vi "Line_detector_Labview.vi"() -> ()   [LabVIEW 2021]
uses:
  <vilib>/Analysis/NI_AALPro.lvlib
  <vilib>/Analysis/8numeric.llb/1D Numeric Integration.vi
  <vilib>/Utility/file.llb/Write To Spreadsheet File (DBL).vi
panel:
  in  "length droplet 13":i32=50
  in  "start droplet 13":i32=885
  in  "length droplet 12":i32=50
  in  "start droplet 12":i32=820
  in  "Length droplet 11":i32=50
  in  "start droplet 11":i32=750
  in  "droplet length 10":i32=50
  in  "start droplet 10":i32=690
  in  "length droplet 9":i32=50
  in  "start droplet 9":i32=630
  in  "length droplet 8":i32=50
  in  "start droplet 8":i32=540
  in  "length droplet 7":i32=50
  in  "start droplet 7":i32=480
  in  "Length droplet 6":i32=50
  in  "start droplet 6":i32=420
  in  "droplet length 5":i32=50
  in  "start droplet 5":i32=380
  out "Waveform Chart":dynamicdata(graph)
  in  "length droplet 4":i32=50
  in  "start droplet 4":i32=315
  in  "length droplet 3":i32=50
  in  "start droplet 3":i32=250
  in  "Length droplet 2":i32=50
  in  "start droplet 2":i32=190
  in  "stop":bool
  in  "droplet length 1":i32=50
  in  "start droplet 1":i32=120
  out "Device Status":i32
  in  "filename":string="CCS_1"
  in  "Directory 2":path=path "C:/My_directory"
  in  "Recording time":dbl=600.0
  out "Time (s)":u32
  out "Waveform Graph":dbl[](graph)=[0.04596838682352941, 0.044503448, 0.04074093858823529, 0.042205794117647064, 0.04124974823529412, 0.03858205317647059, 0.037749302352941175, 0.03488108894117647, 0.033539547999999995, 0.03310773858823529, 0.03099518376470588, 0.03062508070588235, 0.029792362823529414, 0.029021289882352943, 0.028651227529411762, 0.028327385882352937, 0.02806527694117647, 0.026353570588235294, 0.024950359294117645, 0.024194783294117644, 0.024888626823529412, 0.02279143505882353, 0.01915227411764706, 0.019090585411764706, 0.019861556235294116, 0.016870007294117646, 0.01774893270588235, 0.01762559105882353, 0.017687284705882354, 0.016484475294117645, 0.016422783529411764, 0.014063474117647058, 0.012984044, 0.012860665647058823, 0.013492896235294117, 0.013431210352941177, 0.01241350588235294, 0.01182750894117647, 0.01323074917647059, 0.011827489411764706, 0.012212996235294118, 0.010948565176470589, 0.011580750117647058, 0.010115838352941177, 0.009483607764705882, 0.010948526352941176, 0.009730326823529412, 0.011580742352941176, 0.010686367764705882, 0.008018671764705882, 0.008327067764705882, 0.009421913176470589, 0.007879864470588235, 0.008913025176470588, 0.007633115529411765, 0.008650876235294118, 0.008465824705882353, 0.007247633882352941, 0.007124262352941176, 0.007448086117647058, 0.007633124235294117, 0.006862113411764706, 0.008018615529411764, 0.007818177647058822, 0.007370949176470587, 0.0066770442352941176, 0.006044822352941176, 0.006044839058823529, 0.004518220235294117, 0.005273821411764706, 0.005397161882352941, 0.0049654002352941175, 0.005906044235294118, 0.006800401411764707, 0.005212110352941177, 0.004888289176470589, 0.005474254352941177, 0.004888291294117647, 0.004826613176470589, 0.005273799058823529, 0.003932234588235294, 0.004965389411764706, 0.0052737776470588235, 0.0042560430588235295, 0.004826618117647058, 0.004764921647058824, 0.004518198823529412, 0.004071016705882353, 0.003562158823529412, 0.005212115294117647, 0.004518176470588235, 0.00393222305882353, 0.003238310588235294, 0.0033616665882352944, 0.0023439329411764705, 0.003623792, 0.0037471715294117645, 0.002729438823529412, 0.004256026588235294, 0.003932192, 0.003114934117647059, 0.0023439136470588236, 0.0032999837647058826, 0.0031766101176470586, 0.0026060604705882354, 0.0036238037647058825, 0.002991563529411765, 0.003053236470588235, 0.0022822237647058823, 0.0018350458823529411, 0.002729402823529412, 0.0022205331764705884, 0.0023439037647058824, 0.0017116750588235293, 0.0017116759999999999, 0.0015883258823529412, 0.0017733590588235293, 0.001650004, 0.0013878541176470588, 0.001526629411764706, 0.003176581882352941, 0.0013878454117647058, 0.0026060496470588232, 0.0017733687058823528, 0.0017116644705882354, 0.0010794367058823528, 0.0008172868235294117, 0.001141120705882353, 0.0009406536470588235, 0.0013261691764705882, 0.0005705670588235294, 0.0008789717647058824, 0.0015266265882352941, 0.0010177442352941176, 0.0020971644705882354, 0.0018350369411764707, 0.0018350235294117647, 0.003238283294117647, 0.0021588696470588235, 0.002035527294117647, 0.0029915691764705885, 0.0032999729411764705, 0.0038705197647058826, 0.003238293882352941, 0.004132664705882353, 0.003114944705882353, 0.0025443882352941174, 0.004009308705882353, 0.002991563529411765, 0.002482720941176471, 0.0021588795294117647, 0.0025443795294117647, 0.001958410588235294, 0.0022205468235294117, 0.0018967228235294118, 0.0014495164705882353, 0.0008789795294117646, 0.00030843082352941176, 0.000570572, 0.0006939134117647059, 0.0003084084705882353, 9.411764705882353e-10, 0.0, 0.00024673035294117647, 0.0, 7.764705882352941e-09, 0.0001233705882352941, 9.411764705882353e-10, 0.0, 2.823529411764706e-09, 0.0008789534117647059, 9.411764705882353e-10, 0.00012336564705882355, 0.0, 0.0, 0.0, 0.0, 0.0, 7.764705882352941e-09, 0.0, 6.168094117647059e-05, 0.0, 6.168094117647059e-05, 0.0, 0.0, 0.0, 4.705882352941176e-09, 0.0003084056470588235, 0.0004317665882352942, 0.0, 3.764705882352941e-09, 0.00043176847058823533, 0.0, 0.0, 0.0, 0.00012336188235294117, 0.0, 0.0020354865882352942, 0.003500441882352941, 0.0032382910588235293, 0.004009335764705882, 0.004194385411764706, 0.005088741647058824, 0.0048883, 0.007062552235294117, 0.006738748705882354, 0.007694783764705883, 0.0054743, 0.007571457882352942, 0.006800442117647058, 0.007879898588235294, 0.007509780705882353, 0.008141981176470588, 0.0070625724705882355, 0.005597652235294117, 0.004703261882352941, 0.004194387529411765, 0.0031149524705882353, 0.0018967324705882354, 0.0008172889411764706, 0.0, 0.0, 0.0, 0.0, 0.0, 0.0, 0.0, 0.0, 0.0, 0.0, 0.0, 0.0, 0.0, 0.0, 0.0, 0.0, 0.0, 0.0, 0.0, 0.0, 0.0, 0.0, 0.0, 0.0, 0.0, 0.0, 0.0, 0.0, 0.0, 0.0, 0.0, 0.0, 0.0, 0.0, 0.0, 0.0, 0.0, 0.0, 1.2470588235294118e-08, 0.0005705564705882353, 0.0015266061176470588, 0.0022205350588235294, 0.004579854352941177, 0.0033616656470588234, 0.0034233416470588235, 0.00604480494117647, 0.0048883, 0.00610651694117647, 0.00649201505882353, 0.006677062823529412, 0.007370966588235294, 0.006168196941176471, 0.006291567529411765, 0.006430326352941176, 0.0068620832941176475, 0.005721009176470588, 0.005335487764705882, 0.005273805882352941, 0.005273808705882353, 0.004703236705882353, 0.002220570117647059, 0.0017116896470588236, 1.2470588235294118e-08, 0.0, 0.0, 4.705882352941176e-09, 0.0, 0.0, 0.0, 0.0, 0.0, 0.0, 0.0, 0.00012336188235294117, 0.0, 0.0, 0.0, 0.0, 0.0, 0.0, 0.0, 0.0, 0.0, 0.0, 0.0, 0.0, 0.0, 0.0, 0.0, 0.0, 0.0, 0.0, 0.0, 0.0, 0.0, 0.0, 0.0, 0.0, 3.764705882352941e-09, 0.0, 0.00024672376470588235, 0.00043179270588235296, 0.0005705487058823529, 0.0010794211764705883, 0.0004317665882352942, 0.0014495195294117649, 0.0017116750588235293, 0.0023439018823529414, 0.0016500030588235295, 0.0015883025882352942, 0.0018350418823529413, 0.002606044, 0.0010794348235294118, 0.0003701155294117647, 0.000508873411764706, 0.0006939211764705883, 1.4352941176470588e-08, 0.0002467324705882353, 8.705882352941176e-09, 0.0006939115294117647, 9.647058823529411e-09, 0.0, 1.8823529411764705e-09, 0.0, 0.0, 0.0, 6.168094117647059e-05, 0.0, 0.0, 0.0, 0.0, 0.0, 0.0, 0.0, 0.0, 0.0, 0.0, 0.0, 0.0, 0.0, 0.0, 0.0, 0.0, 0.0, 0.0, 0.0, 0.0, 0.0, 0.0, 0.0004317665882352942, 0.0003084047058823529, 4.705882352941176e-09, 0.0008172724705882353, 0.0, 0.0, 0.0004317809411764706, 0.0003084056470588235, 0.0002467247058823529, 0.0006322296470588235, 1.0588235294117647e-08, 1.0588235294117647e-08, 0.0012644689411764707, 0.0016499854117647057, 0.003562113176470588, 0.007571394588235294, 0.010177504705882353, 0.014325583058823529, 0.01622231082352941, 0.016361100705882353, 0.01801109905882353, 0.01902886070588235, 0.021326472941176473, 0.024441421647058825, 0.023932582117647056, 0.02704751223529412, 0.028512411294117645, 0.025906386588235294, 0.02590639058823529, 0.025073692, 0.02195878611764706, 0.02075596494117647, 0.019028845176470587, 0.016361121176470587, 0.012089677176470588, 0.004965434117647059, 0.0017733736470588236, 1.5529411764705883e-08, 0.0008172724705882353, 6.168094117647059e-05, 0.0, 0.0, 0.00037008564705882355, 0.0, 0.0, 0.0, 4.705882352941176e-09, 0.0, 0.0, 0.0, 0.0, 0.0, 0.0, 0.0, 0.0, 0.0, 0.0, 0.0, 0.0, 0.0, 0.0, 0.0, 5.647058823529412e-09, 0.0, 0.0, 0.0, 0.00018504282352941177, 8.705882352941176e-09, 9.411764705882353e-10, 0.0005088696470588235, 4.705882352941176e-09, 0.0, 0.00037008564705882355, 6.168094117647059e-05, 0.0005088677647058824, 0.0012027783529411766, 0.002220532235294118, 0.002035502117647059, 0.0035004564705882354, 0.005273778588235294, 0.004579877882352941, 0.006430301176470588, 0.007062557882352941, 0.005983173647058824, 0.009098046588235294, 0.009545254823529413, 0.008465851764705882, 0.00928313011764706, 0.009421892, 0.008265382117647059, 0.008265373176470588, 0.008327037647058824, 0.006677073411764707, 0.007694804235294118, 0.007370995764705882, 0.007694841176470589, 0.010748057411764706, 0.005983196941176471, 0.004009338823529412, 0.0025444, 0.0015266545882352941, 0.001326154588235294, 0.0, 2.823529411764706e-09, 1.8823529411764705e-09, 0.0, 1.8823529411764705e-09, 0.0, 0.0003084056470588235, 0.00012336188235294117, 2.823529411764706e-09, 0.0003084124705882353, 0.00012336188235294117, 2.023529411764706e-08, 0.0005705487058823529, 0.00030841529411764705, 7.764705882352941e-09, 0.0008172724705882353, 0.0, 7.764705882352941e-09, 1.0588235294117647e-08, 0.0013261498823529411, 0.0005088811764705882, 0.0006322402352941176, 0.0015266303529411765, 0.00152664, 0.0008789776470588235, 0.0015883171764705883, 0.0018350536470588235, 0.002482698588235294, 0.0018967131764705883, 0.003299956470588235, 0.003053241411764706, 0.0033616647058823533, 0.002544370823529412, 0.0037471694117647055, 0.0041943651764705875, 0.005212101647058823, 0.007309279764705882, 0.021326395999999997, 0.0356520414117647, 0.05010099811764706, 0.06888312752941177, 0.09041003435294118, 0.1357459614117647, 0.25250893035294114, 0.4017640254117647, 0.5105091830588235, 0.6714677764705882, 0.747491494117647, 0.8181017988235294, 0.8502693209411765, 0.760615316, 0.7211385315294118, 0.6747849475294118, 0.5846832197647058, 0.37826573882352943, 0.2209918025882353, 0.15752055670588236, 0.09677936094117646, 0.05818176894117647, 0.02749493811764706, 0.01202806611764706, 0.006353262117647059, 0.005474258117647059, 0.004009323294117647, 0.003562127764705882, 0.002482696705882353, 0.002282211294117647, 0.0020971741176470586, 0.0012644941176470587, 0.0010177588235294117, 0.0008789776470588235, 0.0007556089411764706, 0.000570572, 1.9294117647058823e-08, 0.0008172790588235295, 7.764705882352941e-09, 0.0001850524705882353, 6.168188235294118e-05, 0.00018505341176470587, 6.588235294117648e-09, 0.0005705487058823529, 0.00018504470588235293, 0.0006322296470588235, 0.0004317665882352942, 1.6470588235294116e-08, 0.0005705583529411765, 0.0, 0.0007555915294117648, 0.00012336658823529413, 0.00018504282352941177, 8.705882352941176e-09, 6.16875294117647e-05, 6.588235294117648e-09, 0.0005088724705882353, 0.00012336188235294117, 0.0005705487058823529, 0.0005705651764705882, 0.0013878355294117647, 0.006291495764705882, 0.04143446941176471, 0.04633848211764706, 0.04188201364705882, 0.04322355294117647, 0.04627680894117647, 0.04633849952941176, 0.050039426117647064, 0.05213661105882353, 0.05233703811764706, 0.05710188611764706, 0.055899200941176466, 0.0579963734117647, 0.052198324, 0.05341653035294118, 0.050224532, 0.047618446117647054, 0.03876716023529412, 0.032275143058823536, 0.030177897882352943, 0.02704752870588235, 0.024888648235294117, 0.021388202352941175, 0.015651813647058824, 0.01304571811764706, 0.006168240705882353, 0.0028527988235294115, 0.0025443823529411767, 0.0024055905882352942, 0.0027910905882352942, 0.001588300705882353, 0.0017733454117647058, 0.0009406508235294117, 0.0007556070588235294, 0.000308428, 9.647058823529411e-09, 0.00018505341176470587, 0.0, 0.0003084056470588235, 0.0, 0.0, 0.0, 0.00012336188235294117, 0.0, 0.0, 0.0, 0.0, 0.0, 0.0, 9.411764705882353e-10, 0.0, 0.0, 0.0, 0.0, 0.0, 0.0, 0.0, 0.0, 6.168094117647059e-05, 0.0, 7.764705882352941e-09, 0.0003084047058823529, 0.0, 0.00012336188235294117, 0.000632235294117647, 0.004317687058823529, 0.008080301411764707, 0.011765773411764706, 0.014248492470588235, 0.016993331294117647, 0.021125988470588233, 0.019984941647058826, 0.024117611294117648, 0.024888671529411766, 0.027432984235294118, 0.026677430588235292, 0.02602975435294118, 0.023547096470588235, 0.024194724, 0.023608739529411765, 0.022529335764705883, 0.020555484470588237, 0.019414364705882352, 0.016484510352941177, 0.014325638352941178, 0.01056306705882353, 0.007247652235294118, 0.0035004962352941176, 0.001079464, 4.705882352941176e-09, 0.00037008564705882355, 6.588235294117648e-09, 8.705882352941176e-09, 0.0, 0.0, 0.0, 0.0, 6.168094117647059e-05, 0.0, 0.0, 0.0, 0.0, 0.0, 0.0, 0.0, 0.0, 0.0, 0.0, 0.0, 0.0, 0.0, 0.0, 0.0, 0.0, 6.168094117647059e-05, 3.764705882352941e-09, 0.0, 0.0, 9.411764705882353e-10, 0.0, 0.00037008564705882355, 0.0, 0.0, 0.0, 0.0, 0.00037008564705882355, 0.0012027849411764707, 0.003500431294117647, 0.005597629882352941, 0.007124247764705882, 0.007448091058823529, 0.008913033882352941, 0.00865088305882353, 0.011519072, 0.010300879294117646, 0.010563029176470588, 0.012660198588235293, 0.011765825882352941, 0.013616245411764705, 0.011580789882352942, 0.008913071764705882, 0.009606945411764704, 0.008327048470588235, 0.006677063764705883, 0.005906063764705882, 0.005335507294117647, 0.004071030352941177, 0.0028528143529411767, 0.0013878590588235293, 0.0014495176470588236, 0.0, 0.0, 0.0, 0.0, 3.764705882352941e-09, 0.0, 0.0, 0.0, 0.0, 0.0, 0.0, 0.0, 0.0, 0.0, 0.0, 0.0, 0.0, 0.0, 0.0, 0.0, 0.0, 0.0, 0.0, 0.0, 0.0, 0.0, 0.0, 0.0, 0.0, 0.0, 0.0, 0.0, 0.0, 0.0, 0.0, 0.0, 0.0, 0.0, 0.0, 0.0024055623529411767, 0.0034233367058823534, 0.005088728941176471, 0.004965383764705882, 0.004764925411764706, 0.006615369176470588, 0.007000902352941176, 0.006492013176470589, 0.007633104705882353, 0.007185919764705883, 0.009159751764705883, 0.008527517176470588, 0.007124297176470589, 0.007000902352941176, 0.0070008964705882346, 0.0066153682352941175, 0.00502707905882353, 0.004132698823529412, 0.004317728941176471, 0.0035621296470588234, 0.0038705275294117643, 0.0026677317647058824, 1.3411764705882353e-08, 9.411764705882353e-10, 0.0, 0.0, 0.0, 0.0, 0.0, 0.0, 0.0, 0.0, 0.0, 0.0, 0.0, 0.0, 0.0, 0.0, 0.0, 0.0, 0.0, 0.0, 0.0, 0.0, 0.0, 0.0, 0.0, 0.0, 0.0, 0.0, 0.0, 0.0, 0.0, 1.8823529411764705e-09, 0.0, 0.0, 0.0, 0.0, 0.0, 0.0, 0.0, 0.0, 0.0006939105882352941, 0.0014495185882352941, 0.0020971548235294117, 0.002035489411764706, 0.0026060545882352943, 0.004194354352941176, 0.003623829882352941, 0.003932212235294118, 0.005027058823529412, 0.004071014823529412, 0.004826601647058824, 0.0038088543529411763, 0.0037471684705882354, 0.003747174352941177, 0.0032999856470588237, 0.004009318352941176, 0.0034233367058823534, 0.002606061411764706, 0.0017733482352941176, 0.0008789804705882352, 2.1176470588235293e-08, 0.0, 1.8823529411764705e-09, 0.0, 0.0, 0.0, 0.0, 0.0003084047058823529, 0.0, 0.0, 0.0, 0.0, 0.0, 0.0, 0.0, 0.0, 0.0, 0.0, 0.0, 0.0, 0.0, 0.0, 0.0, 0.0, 0.0, 0.0, 0.0, 0.0, 0.0, 0.0, 0.0, 0.0, 0.0, 0.0, 0.0, 0.0, 0.0, 0.0, 0.00012336188235294117, 0.0, 0.0, 0.0, 0.0008789611764705882, 0.0017116750588235293, 0.0029144574117647057, 0.0032382910588235293, 0.004579859294117647, 0.004317732705882353, 0.004518185176470588, 0.004826578117647059, 0.003932218117647058, 0.00539715905882353, 0.0057209672941176464, 0.005397158117647059, 0.004456525647058823, 0.004009320235294118, 0.004071015764705883, 0.003685487529411765, 0.004317724941176471, 0.0031149291764705884, 0.0025443969411764705, 0.003361657882352941, 0.0018967200000000002, 0.001017760705882353, 0.0003700934117647059, 0.0, 0.0, 0.0, 0.0, 0.0, 0.0, 0.00018504282352941177, 0.0, 2.823529411764706e-09, 0.0, 0.00018504658823529412, 0.00024672376470588235, 5.647058823529412e-09, 0.0, 0.0, 0.00012336188235294117, 0.0, 0.0, 6.168094117647059e-05, 0.0, 0.0005705611764705883, 0.00012336188235294117, 3.764705882352941e-09, 0.0, 6.588235294117648e-09, 0.0, 0.0006939162352941177, 0.0, 0.0004317665882352942, 0.0, 0.0, 9.411764705882353e-10, 1.5529411764705883e-08, 0.001141108, 6.170211764705882e-05, 0.0013261489411764706, 0.0005705602352941176, 0.0006322296470588235, 0.0006939171764705882, 0.000878972705882353, 0.000632244, 0.0019583872941176467, 0.0018350322352941176, 0.002544393176470588, 0.003747145176470588, 0.0026677482352941177, 0.002991556705882353, 0.004070993411764706, 0.0037471470588235295, 0.004379393411764705, 0.0041943418823529414, 0.003176631529411765, 0.0030532609411764704, 0.0036854943529411764, 0.005597627764705882, 0.004641558823529412, 0.005088735764705882, 0.006862099764705883, 0.004071012000000001, 0.0022822520000000002, 0.002991570117647059, 0.0024826889411764708, 0.0018350536470588235, 0.002606063294117647, 0.002667734588235294, 0.0024056051764705885, 0.0025443717647058825, 0.0021588736470588236, 0.0019583941176470588, 0.0023439164705882356, 0.002282245176470588, 0.0018967101176470588, 0.002282243294117647, 0.0027910945882352943, 0.0019584056470588235, 0.0020971762352941176, 0.001896724705882353, 0.0023438990588235294, 0.0024826821176470587, 0.0012028025882352942, 0.0012644776470588234, 0.0032382804705882355, 0.00043179270588235296, 0.001079451294117647, 0.0015266322352941177, 0.002158864, 0.0011411129411764706, 0.0015266275294117649, 0.0015883063529411766, 0.0024826830588235292, 0.002544364, 0.0017116672941176472, 0.001588300705882353, 0.0007556235294117647, 0.001958396, 0.0009406595294117647, 0.0016499795294117648, 0.0012027995294117647, 0.001141116705882353, 0.0010177635294117647, 0.0012028016470588237, 0.002405581882352941, 0.0013878531764705882, 0.0024826781176470586, 0.0021588590588235293, 0.0015883103529411764, 0.002991547764705882, 0.002158849411764706, 0.002220536, 0.0018967150588235294, 0.0019584009411764704, 0.00248268, 0.0022205710588235296, 0.002343919294117647, 0.0030532609411764704, 0.002667718117647059, 0.002544368705882353, 0.002606047764705882, 0.003685469176470588, 0.0, 0.0, 0.0, 0.0, 0.0, 0.0, 0.0, 0.0, 0.0, 0.0, 0.0, 0.0, 0.0, 0.0, 0.0, 0.0, 0.0, 0.0, 0.0, 0.0, 0.0, 0.0, 0.0, 0.0, 0.0, 0.0, 0.0, 0.0, 0.0, 0.0, 0.0, 0.0, 0.0, 0.0, 0.0, 0.0, 0.0, 0.0, 0.0, 0.0, 0.0, 0.0, 0.0, 0.0, 0.0, 0.0, 0.0, 0.0, 0.0, 0.0, 0.0, 0.0, 0.0, 0.0, 0.0, 0.0, 0.0, 0.0, 0.0, 0.0, 0.0, 0.0, 0.0, 0.0, 0.0, 0.0, 0.0, 0.0, 0.0, 0.0, 0.0, 0.0, 0.0, 0.0, 0.0, 0.0, 0.0, 0.0, 0.0, 0.0, 0.0, 0.0, 0.0, 0.0, 0.0, 0.0, 0.0, 0.0, 0.0, 0.0, 0.0, 0.0, 0.0, 0.0, 0.0, 0.0, 0.0, 0.0, 0.0, 0.0, 0.0, 0.0, 0.0, 0.0, 0.0, 0.0, 0.0, 0.0, 0.0, 0.0, 0.0, 0.0, 0.0, 0.0, 0.0, 0.0, 0.0, 0.0, 0.0, 0.0, 0.0, 0.0, 0.0, 0.0, 0.0, 0.0, 0.0, 0.0, 0.0, 0.0, 0.0, 0.0, 0.0, 0.0, 0.0, 0.0, 0.0, 0.0, 0.0, 0.0, 0.0, 0.0, 0.0, 0.0, 0.0, 0.0, 0.0, 0.0, 0.0, 0.0, 0.0, 0.0, 0.0, 0.0, 0.0, 0.0, 0.0, 0.0, 0.0, 0.0, 0.0, 0.0, 0.0, 0.0, 0.0, 0.0, 0.0, 0.0, 0.0, 0.0, 0.0, 0.0, 0.0, 0.0, 0.0, 0.0, 0.0, 0.0, 0.0, 0.0, 0.0, 0.0, 0.0, 0.0, 0.0, 0.0, 0.0, 0.0, 0.0, 0.0, 0.0, 0.0, 0.0, 0.0, 0.0, 0.0, 0.0, 0.0, 0.0, 0.0, 0.0, 0.0, 0.0, 0.0, 0.0, 0.0, 0.0, 0.0, 0.0, 0.0, 0.0, 0.0, 0.0, 0.0, 0.0, 0.0, 0.0, 0.0, 0.0, 0.0, 0.0, 0.0, 0.0, 0.0, 0.0, 0.0, 0.0, 0.0, 0.0, 0.0, 0.0, 0.0, 0.0, 0.0, 0.0, 0.0, 0.0, 0.0, 0.0, 0.0, 0.0, 0.0, 0.0, 0.0, 0.0, 0.0, 0.0, 0.0, 0.0, 0.0, 0.0, 0.0, 0.0, 0.0, 0.0, 0.0, 0.0, 0.0, 0.0, 0.0, 0.0, 0.0, 0.0, 0.0, 0.0, 0.0, 0.0, 0.0, 0.0, 0.0, 0.0, 0.0, 0.0, 0.0, 0.0, 0.0, 0.0, 0.0, 0.0, 0.0, 0.0, 0.0, 0.0, 0.0, 0.0, 0.0, 0.0, 0.0, 0.0, 0.0, 0.0, 0.0, 0.0, 0.0, 0.0, 0.0, 0.0, 0.0, 0.0, 0.0, 0.0, 0.0, 0.0, 0.0, 0.0, 0.0, 0.0, 0.0, 0.0, 0.0, 0.0, 0.0, 0.0, 0.0, 0.0, 0.0, 0.0, 0.0, 0.0, 0.0, 0.0, 0.0, 0.0, 0.0, 0.0, 0.0, 0.0, 0.0, 0.0, 0.0, 0.0, 0.0, 0.0, 0.0, 0.0, 0.0, 0.0, 0.0, 0.0, 0.0, 0.0, 0.0, 0.0, 0.0, 0.0, 0.0, 0.0, 0.0, 0.0, 0.0, 0.0, 0.0, 0.0, 0.0, 0.0, 0.0, 0.0, 0.0, 0.0, 0.0, 0.0, 0.0, 0.0, 0.0, 0.0, 0.0, 0.0, 0.0, 0.0, 0.0, 0.0, 0.0, 0.0, 0.0, 0.0, 0.0, 0.0, 0.0, 0.0, 0.0, 0.0, 0.0, 0.0, 0.0, 0.0, 0.0, 0.0, 0.0, 0.0, 0.0, 0.0, 0.0, 0.0, 0.0, 0.0, 0.0, 0.0, 0.0, 0.0, 0.0, 0.0, 0.0, 0.0, 0.0, 0.0, 0.0, 0.0, 0.0, 0.0, 0.0, 0.0, 0.0, 0.0, 0.0, 0.0, 0.0, 0.0, 0.0, 0.0, 0.0, 0.0, 0.0, 0.0, 0.0, 0.0, 0.0, 0.0, 0.0, 0.0, 0.0, 0.0, 0.0, 0.0, 0.0, 0.0, 0.0, 0.0, 0.0, 0.0, 0.0, 0.0, 0.0, 0.0, 0.0, 0.0, 0.0, 0.0, 0.0, 0.0, 0.0, 0.0, 0.0, 0.0, 0.0, 0.0, 0.0, 0.0, 0.0, 0.0, 0.0, 0.0, 0.0, 0.0, 0.0, 0.0, 0.0, 0.0, 0.0, 0.0, 0.0, 0.0, 0.0, 0.0, 0.0, 0.0, 0.0, 0.0, 0.0, 0.0, 0.0, 0.0, 0.0, 0.0, 0.0, 0.0, 0.0, 0.0, 0.0, 0.0, 0.0, 0.0, 0.0, 0.0, 0.0, 0.0, 0.0, 0.0, 0.0, 0.0, 0.0, 0.0, 0.0, 0.0, 0.0, 0.0, 0.0, 0.0, 0.0, 0.0, 0.0, 0.0, 0.0, 0.0, 0.0, 0.0, 0.0, 0.0, 0.0, 0.0, 0.0, 0.0, 0.0, 0.0, 0.0, 0.0, 0.0, 0.0, 0.0, 0.0, 0.0, 0.0, 0.0, 0.0, 0.0, 0.0, 0.0, 0.0, 0.0, 0.0, 0.0, 0.0, 0.0, 0.0, 0.0, 0.0, 0.0, 0.0, 0.0, 0.0, 0.0, 0.0, 0.0, 0.0, 0.0, 0.0, 0.0, 0.0, 0.0, 0.0, 0.0, 0.0, 0.0, 0.0, 0.0, 0.0, 0.0, 0.0, 0.0, 0.0, 0.0, 0.0, 0.0, 0.0, 0.0, 0.0, 0.0, 0.0, 0.0, 0.0, 0.0, 0.0, 0.0, 0.0, 0.0, 0.0, 0.0, 0.0, 0.0, 0.0, 0.0, 0.0, 0.0, 0.0, 0.0, 0.0, 0.0, 0.0, 0.0, 0.0, 0.0, 0.0, 0.0, 0.0, 0.0, 0.0, 0.0, 0.0, 0.0, 0.0, 0.0, 0.0, 0.0, 0.0, 0.0, 0.0, 0.0, 0.0, 0.0, 0.0, 0.0, 0.0, 0.0, 0.0, 0.0, 0.0, 0.0, 0.0, 0.0, 0.0, 0.0, 0.0, 0.0, 0.0, 0.0, 0.0, 0.0, 0.0, 0.0, 0.0, 0.0, 0.0, 0.0, 0.0, 0.0, 0.0, 0.0, 0.0, 0.0, 0.0, 0.0, 0.0, 0.0, 0.0, 0.0, 0.0, 0.0, 0.0, 0.0, 0.0, 0.0, 0.0, 0.0, 0.0, 0.0, 0.0, 0.0, 0.0, 0.0, 0.0, 0.0, 0.0, 0.0, 0.0, 0.0, 0.0, 0.0, 0.0, 0.0, 0.0, 0.0, 0.0, 0.0, 0.0, 0.0, 0.0, 0.0, 0.0, 0.0, 0.0, 0.0, 0.0, 0.0, 0.0, 0.0, 0.0, 0.0, 0.0, 0.0, 0.0, 0.0, 0.0, 0.0, 0.0, 0.0, 0.0, 0.0, 0.0, 0.0, 0.0, 0.0, 0.0, 0.0, 0.0, 0.0, 0.0, 0.0, 0.0, 0.0, 0.0, 0.0, 0.0, 0.0, 0.0, 0.0, 0.0, 0.0, 0.0, 0.0, 0.0, 0.0, 0.0, 0.0, 0.0, 0.0, 0.0, 0.0, 0.0, 0.0, 0.0, 0.0, 0.0, 0.0, 0.0, 0.0, 0.0, 0.0, 0.0, 0.0, 0.0, 0.0, 0.0, 0.0, 0.0, 0.0, 0.0, 0.0, 0.0, 0.0, 0.0, 0.0, 0.0, 0.0, 0.0, 0.0, 0.0, 0.0, 0.0, 0.0, 0.0, 0.0, 0.0, 0.0, 0.0, 0.0, 0.0, 0.0, 0.0, 0.0, 0.0, 0.0, 0.0, 0.0, 0.0, 0.0, 0.0, 0.0, 0.0, 0.0, 0.0, 0.0, 0.0, 0.0, 0.0, 0.0, 0.0, 0.0, 0.0, 0.0, 0.0, 0.0, 0.0, 0.0, 0.0, 0.0, 0.0, 0.0, 0.0, 0.0, 0.0, 0.0, 0.0, 0.0, 0.0, 0.0, 0.0, 0.0, 0.0, 0.0, 0.0, 0.0, 0.0, 0.0, 0.0, 0.0, 0.0, 0.0, 0.0, 0.0, 0.0, 0.0, 0.0, 0.0, 0.0, 0.0, 0.0, 0.0, 0.0, 0.0, 0.0, 0.0, 0.0, 0.0, 0.0, 0.0, 0.0, 0.0, 0.0, 0.0, 0.0, 0.0, 0.0, 0.0, 0.0, 0.0, 0.0, 0.0, 0.0, 0.0, 0.0, 0.0, 0.0, 0.0, 0.0, 0.0, 0.0, 0.0, 0.0, 0.0, 0.0, 0.0, 0.0, 0.0, 0.0, 0.0, 0.0, 0.0, 0.0, 0.0, 0.0, 0.0, 0.0, 0.0, 0.0, 0.0, 0.0, 0.0, 0.0, 0.0, 0.0, 0.0, 0.0, 0.0, 0.0, 0.0, 0.0, 0.0, 0.0, 0.0, 0.0, 0.0, 0.0, 0.0, 0.0, 0.0, 0.0, 0.0, 0.0, 0.0, 0.0, 0.0, 0.0, 0.0, 0.0, 0.0, 0.0, 0.0, 0.0, 0.0, 0.0, 0.0, 0.0, 0.0, 0.0, 0.0, 0.0, 0.0, 0.0, 0.0, 0.0, 0.0, 0.0, 0.0, 0.0, 0.0, 0.0, 0.0, 0.0, 0.0, 0.0, 0.0, 0.0, 0.0, 0.0, 0.0, 0.0, 0.0, 0.0, 0.0, 0.0, 0.0, 0.0, 0.0, 0.0, 0.0, 0.0, 0.0, 0.0, 0.0, 0.0, 0.0, 0.0, 0.0, 0.0, 0.0, 0.0, 0.0, 0.0, 0.0, 0.0, 0.0, 0.0, 0.0, 0.0, 0.0, 0.0, 0.0, 0.0, 0.0, 0.0, 0.0, 0.0, 0.0, 0.0, 0.0, 0.0, 0.0, 0.0, 0.0, 0.0, 0.0, 0.0, 0.0, 0.0, 0.0, 0.0, 0.0, 0.0, 0.0, 0.0, 0.0, 0.0, 0.0, 0.0, 0.0, 0.0, 0.0, 0.0, 0.0, 0.0, 0.0, 0.0, 0.0, 0.0, 0.0, 0.0, 0.0, 0.0, 0.0, 0.0, 0.0, 0.0, 0.0, 0.0, 0.0]
  in  "Integration Time (ms)":dbl=5.0
  out "FPS":dbl
  out "CCS100 Resource name":string[](array[string])
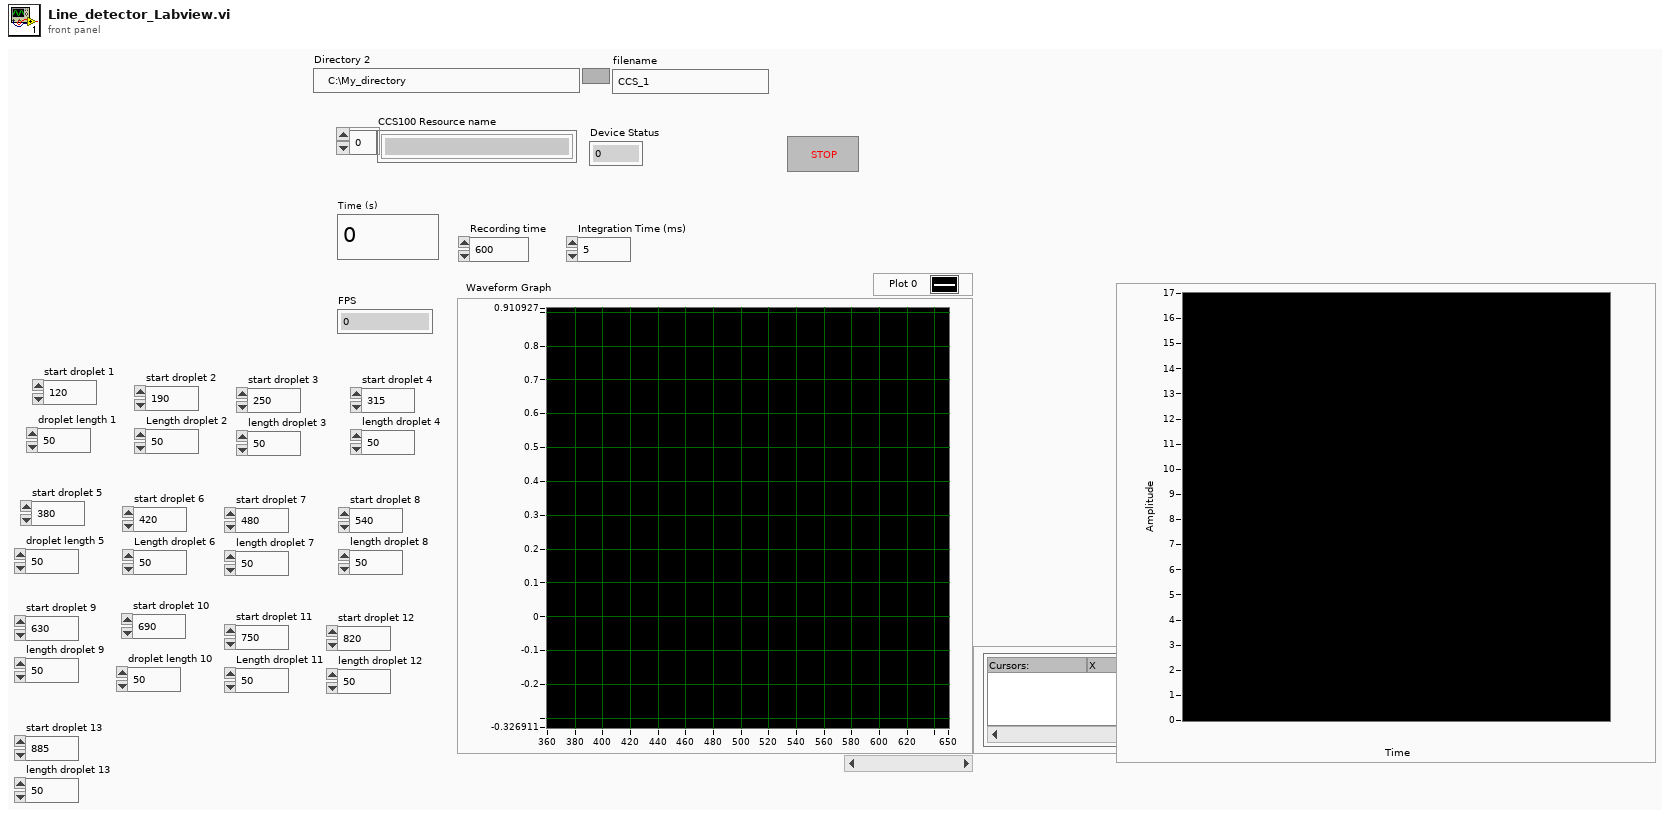
[diagram p1: front panel]
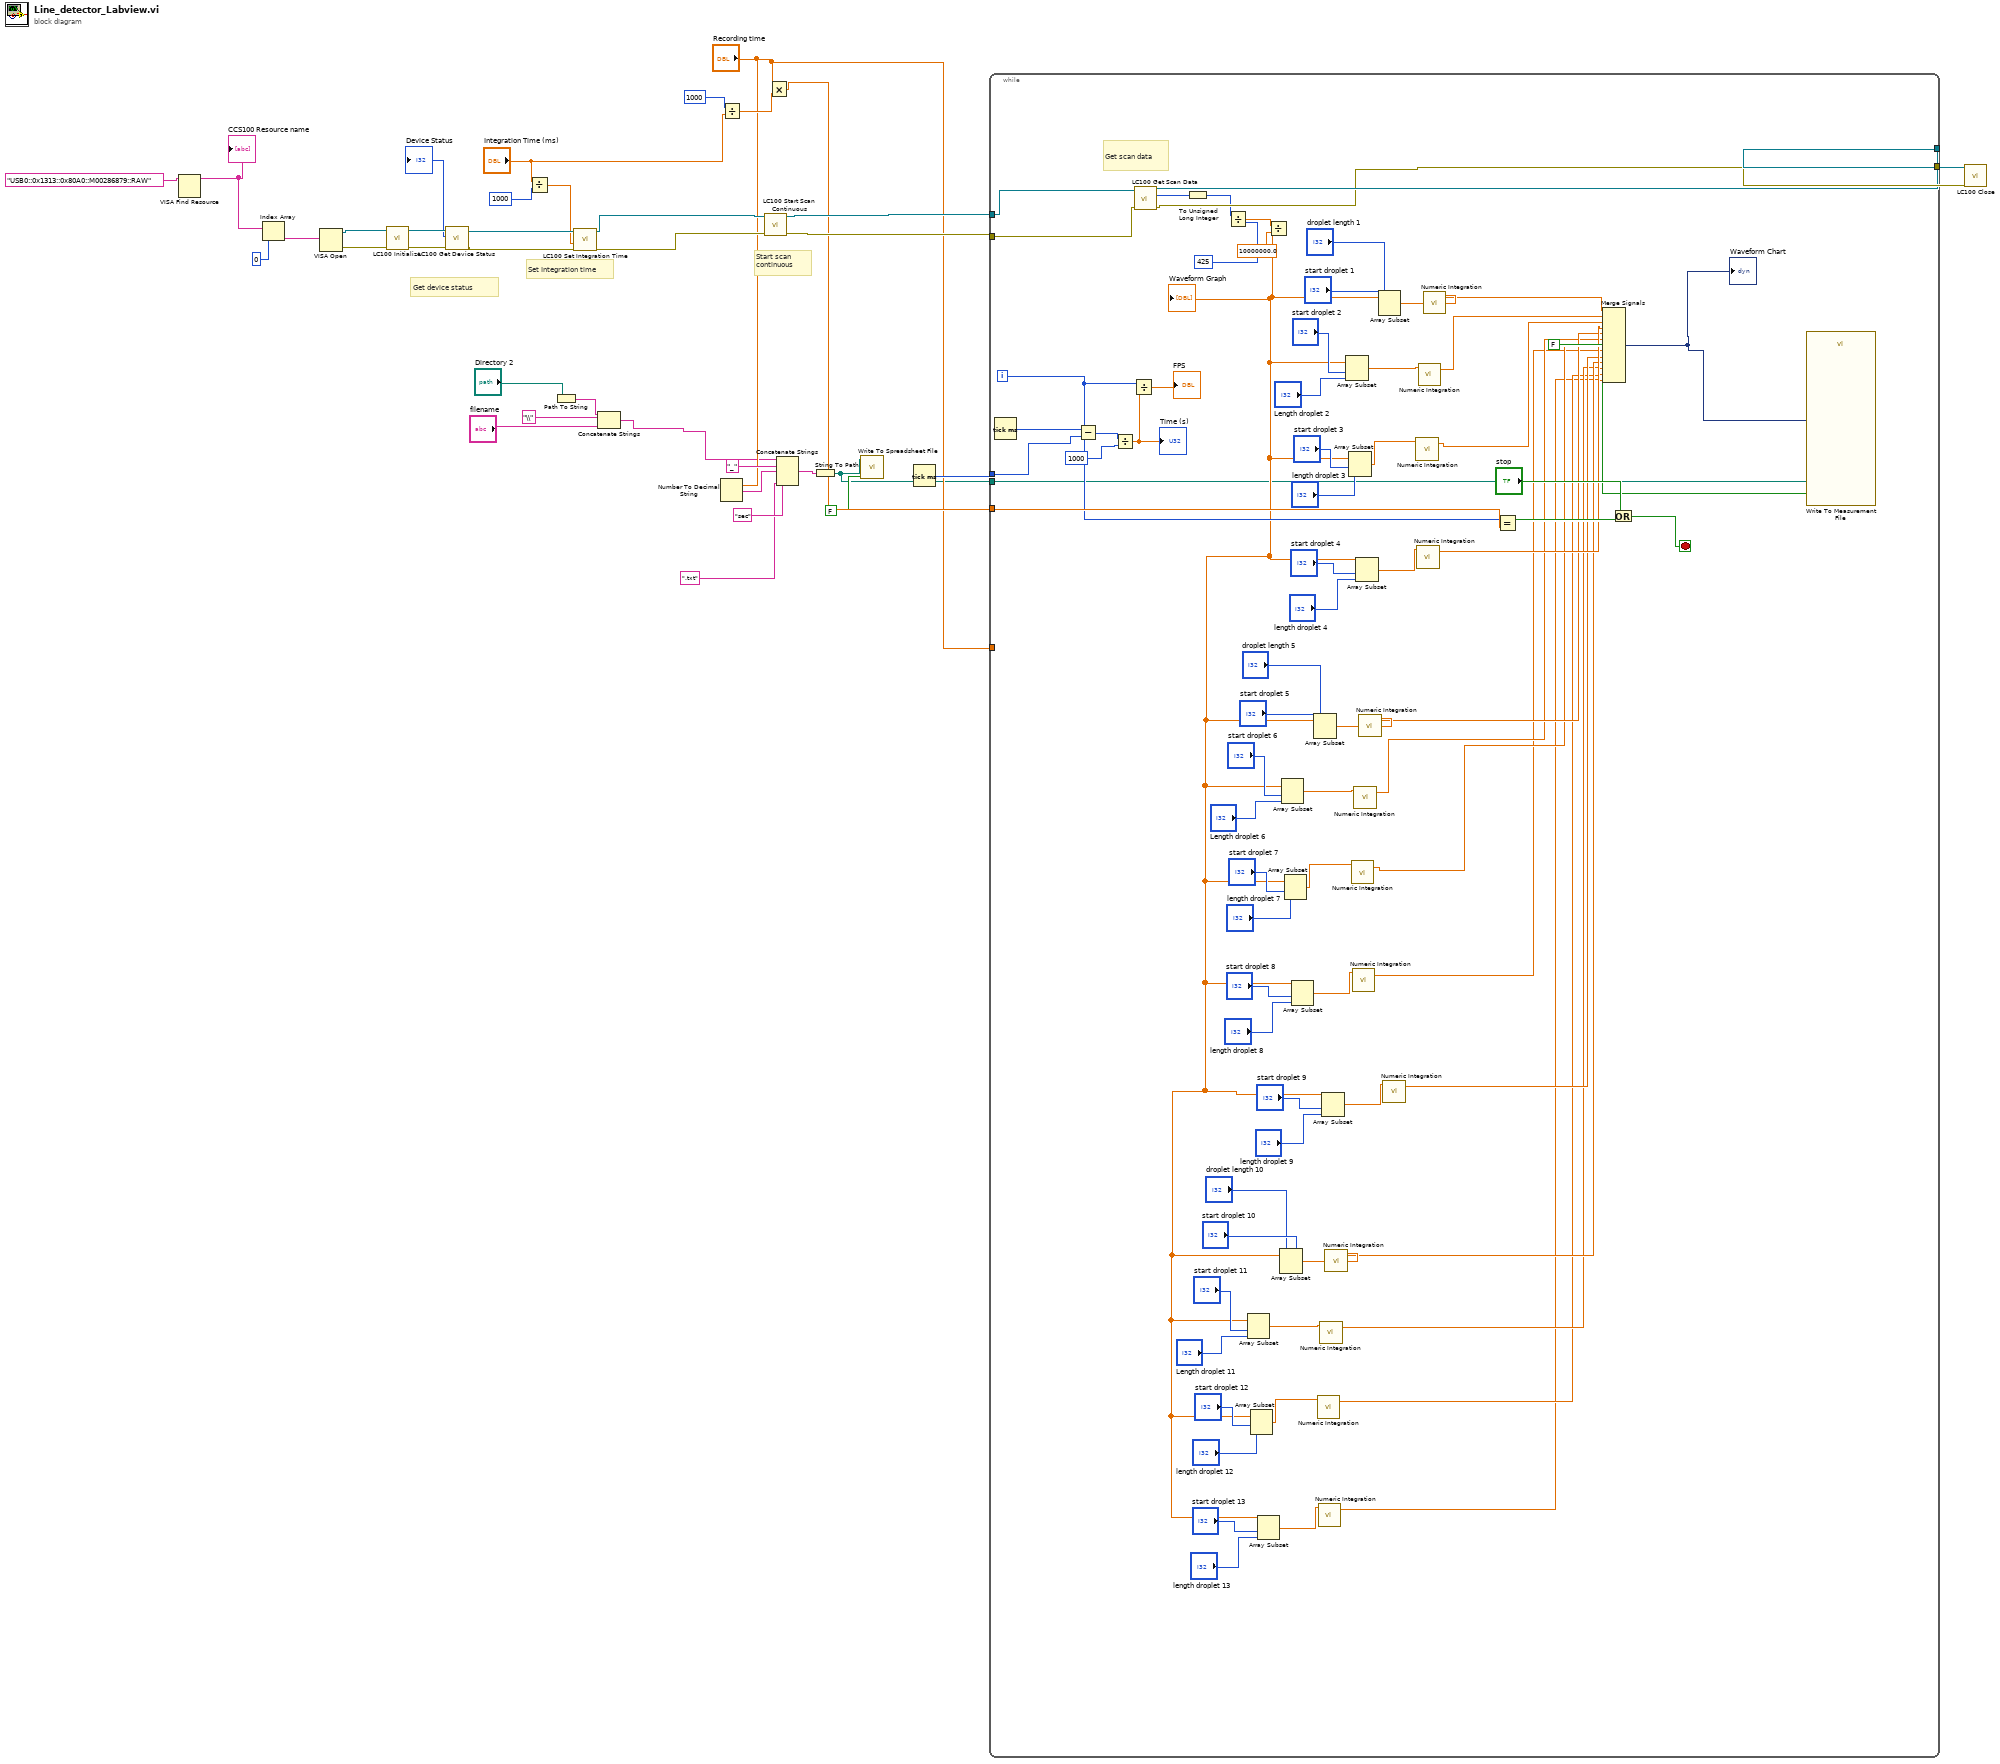
[diagram p0: block diagram]
diagram:
  # "Start scan continuous"
  # "Set Integration time"
  # "Get device status"
  n1 = VISA Find Resource(11:"USB0::0x1313::0x80A0::M00286879::RAW") -> (3:w36:string[])  [unwired: 2 in, 2 out]
  "CCS100 Resource name" <- w36
  n2 = Index Array(array=w36, index=0) -> (element=w25:string)
  n3 = VISA Open(VISA resource name=w25) -> (VISA resource name=w24:refnum<visa-resource-name>, error out=w23:errorcluster)  [unwired: 4 in]
  n4 = call <instrlib>:"LC100 Initialize.vi"("error in (no error)"=w23, "resource name"=w24) -> ("error out"=w21:errorcluster, "instrument handle out"=w22:refnum<visa-resource-name>)  [unwired: 8 in]
  n5 = call <instrlib>:"LC100 Get Device Status.vi"("error in (no error)"=w21, "instrument handle"=w22) -> ("error out"=w18:errorcluster, "Device Status"=→"Device Status":i32, "instrument handle out"=w19:refnum<visa-resource-name>)  [unwired: 7 in]
  n6 = Divide(x="Integration Time (ms)", y=1000) -> (x/y=w17:dbl)
  n7 = Path To String(path="Directory 2") -> (string=w27:string)
  n8 = call <instrlib>:"LC100 Set Integration Time.vi"("error in (no error)"=w18, "Integration Time [s] (0.00105)"=w17, "instrument handle"=w19) -> ("error out"=w13:errorcluster, "instrument handle out"=w16:refnum<visa-resource-name>)  [unwired: 7 in]
  n9 = Concatenate Strings(w27, "\\", "filename") -> (w2:string)
  n10 = Number To Decimal String(number="Recording time") -> (decimal integer string=w6:string)  [unwired: 1 in]
  n11 = Divide(x=1000, y="Integration Time (ms)") -> (x/y=w30:dbl)
  n12 = call <instrlib>:"LC100 Start Scan Continuous.vi"("error in (no error)"=w13, "instrument handle"=w16) -> ("error out"=w14:errorcluster, "instrument handle out"=w15:refnum<visa-resource-name>)  [unwired: 8 in]
  n13 = Multiply(x="Recording time", y=w30) -> (x*y=w10:dbl)
  n14 = Concatenate Strings(w2, "_", w6, "sec", ".txt") -> (w7:string)
  n15 = String To Path(string=w7) -> (path=w3:path)
  n16 = call-poly <vilib>:"Write To Spreadsheet File.vi"("append to file? (new file:F)"=FALSE, "file path (dialog if empty)"=w3) -> ()  [unwired: 4 in, 3 out]
  n17 = Tick Count (ms)() -> (millisecond timer value=w34:u32)
  n18 = while {
    tunnel: [w106] -> w12
    tunnel: [w105] -> w11
    tunnel: w34 -> [w110]
    tunnel: w14 -> [w107]
    tunnel: w15 -> [w108]
    tunnel: w10 -> [w84]
    tunnel: "Recording time" -> [_]
    tunnel: w3 -> [w40]
    i -> [w83]
    stop <- w100 stop-if-true
    # "Get scan data"
    n19 = Tick Count (ms)() -> (millisecond timer value=w111:u32)
    n20 = Subtract(x=w111, y=w110) -> (x-y=w112:u32)
    n21 = Divide(x=w112, y=u32 1000) -> (x/y=w41:dbl)
    "Time (s)" <- w41
    n22 = Divide(x=w83, y=w41) -> (x/y=→"FPS":dbl)
    n23 = call <instrlib>:"LC100 Get Scan Data.vi"("error in (no error)"=w107, "instrument handle"=w108) -> ("error out"=w105:errorcluster, "Data"=w39:u32[], "instrument handle out"=w106:refnum<visa-resource-name>)  [unwired: 7 in]
    n24 = To Unsigned Long Integer(number=w39) -> (unsigned 32bit integer=w38:u32[])
    n25 = Divide(x=w38, y=425) -> (x/y=w43:dbl[])
    n26 = Divide(x=w43, y=10000000.0) -> (x/y=w42:dbl[])
    "Waveform Graph" <- w42
    n27 = Array Subset(array=w42, index="start droplet 11", length="Length droplet 11") -> (w58:dbl[])
    n28 = Array Subset(array=w42, index="start droplet 12", length="length droplet 12") -> (w55:dbl[])
    n29 = Array Subset(array=w42, index="start droplet 13", length="length droplet 13") -> (w52:dbl[])
    n30 = Array Subset(array=w42, index="start droplet 10", length="droplet length 10") -> (w61:dbl[])
    n31 = Array Subset(array=w42, index="start droplet 6", length="Length droplet 6") -> (w77:dbl[])
    n32 = Array Subset(array=w42, index="start droplet 7", length="length droplet 7") -> (w74:dbl[])
    n33 = Array Subset(array=w42, index="start droplet 8", length="length droplet 8") -> (w71:dbl[])
    n34 = Array Subset(array=w42, index="start droplet 5", length="droplet length 5") -> (w80:dbl[])
    n35 = call-poly <vilib>:"Numeric Integration.vi"("Input Array"=w55) -> ("result"=w48:dbl)  [unwired: 2 in, 1 out]
    n36 = call-poly <vilib>:"Numeric Integration.vi"("Input Array"=w52) -> ("result"=w47:dbl)  [unwired: 2 in, 1 out]
    n37 = call-poly <vilib>:"Numeric Integration.vi"("Input Array"=w58) -> ("result"=w49:dbl)  [unwired: 2 in, 1 out]
    n38 = Array Subset(array=w42, index="start droplet 9", length="length droplet 9") -> (w64:dbl[])
    n39 = call-poly <vilib>:"Numeric Integration.vi"("Input Array"=w61) -> ("result"=w50:dbl)  [unwired: 2 in, 1 out]
    n40 = Array Subset(array=w42, index="start droplet 2", length="Length droplet 2") -> (w96:dbl[])
    n41 = Array Subset(array=w42, index="start droplet 3", length="length droplet 3") -> (w90:dbl[])
    n42 = call-poly <vilib>:"Numeric Integration.vi"("Input Array"=w74) -> ("result"=w68:dbl)  [unwired: 2 in, 1 out]
    n43 = call-poly <vilib>:"Numeric Integration.vi"("Input Array"=w71) -> ("result"=w67:dbl)  [unwired: 2 in, 1 out]
    n44 = call-poly <vilib>:"Numeric Integration.vi"("Input Array"=w77) -> ("result"=w69:dbl)  [unwired: 2 in, 1 out]
    n45 = Array Subset(array=w42, index="start droplet 4", length="length droplet 4") -> (w86:dbl[])
    n46 = call-poly <vilib>:"Numeric Integration.vi"("Input Array"=w80) -> ("result"=w70:dbl)  [unwired: 2 in, 1 out]
    n47 = Array Subset(array=w42, index="start droplet 1", length="droplet length 1") -> (w99:dbl[])
    n48 = call-poly <vilib>:"Numeric Integration.vi"("Input Array"=w64) -> ("result"=w51:dbl)  [unwired: 2 in, 1 out]
    n49 = call-poly <vilib>:"Numeric Integration.vi"("Input Array"=w90) -> ("result"=w89:dbl)  [unwired: 2 in, 1 out]
    n50 = call-poly <vilib>:"Numeric Integration.vi"("Input Array"=w86) -> ("result"=w85:dbl)  [unwired: 2 in, 1 out]
    n51 = call-poly <vilib>:"Numeric Integration.vi"("Input Array"=w96) -> ("result"=w94:dbl)  [unwired: 2 in, 1 out]
    n52 = call-poly <vilib>:"Numeric Integration.vi"("Input Array"=w99) -> ("result"=w93:dbl)  [unwired: 2 in, 1 out]
    n53 = Equal?(x=w83, y=w84) -> (x = y?=w101:bool)
    n54 = Merge Signals(w93, w94, w89, w85, w70, w69, w68, w67, w51, w50, w49, w48, w47) -> (w45:dynamicdata)
    "Waveform Chart" <- w45
    n55 = Or(x="stop", y=w101) -> (x .or. y?=w100:bool)
    n56 = call "Write To Measurement File"("Signals"=w45, "Reset"=FALSE, "Filename"=w40) -> ()  [unwired: 14 in, 3 out]
  }
  n57 = call <instrlib>:"LC100 Close.vi"("error in (no error)"=w11, "instrument handle"=w12) -> ()  [unwired: 9 in, 1 out]
